vi "Detector Raw Image.vi"(8 "error in (no error)":errorcluster) -> (0 "error out":errorcluster)   [LabVIEW 2018]
uses:
  SesWrapper/SesWrapper.lvlib
panel:
  in  "stop":bool
  out "Camera Image":u8[][](graph)
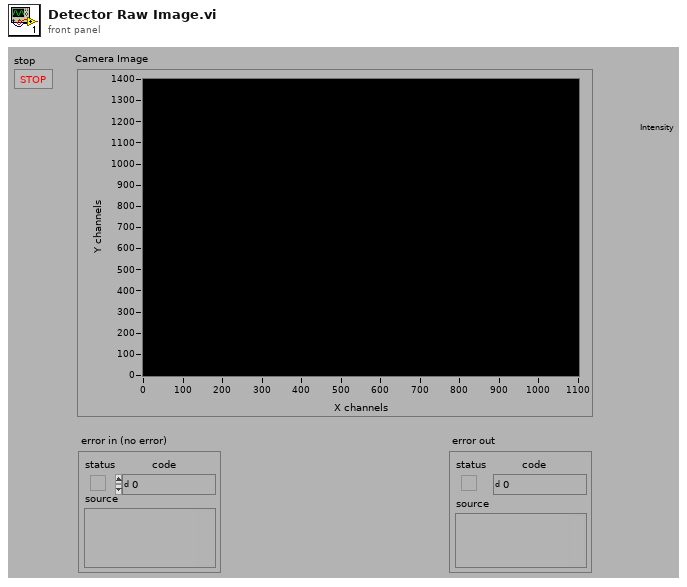
[diagram p1: front panel]
types:
  T1 = cluster{"timerControlled_":u8, "@dummy control@":i8, "@dummy control@":i8, "@dummy control@":i8, "xChannels_":i32, "yChannels_":i32, "maxSlices_":i32, "maxChannels_":i32, "frameRate_":i32, "adcPresent_":u8, "discPresent_":u8}
  T2 = cluster{"timerControlled_":u8, "xChannels_":i32, "yChannels_":i32, "maxSlices_":i32, "maxChannels_":i32, "frameRate_":i32, "adcPresent_":u8, "discPresent_":u8}
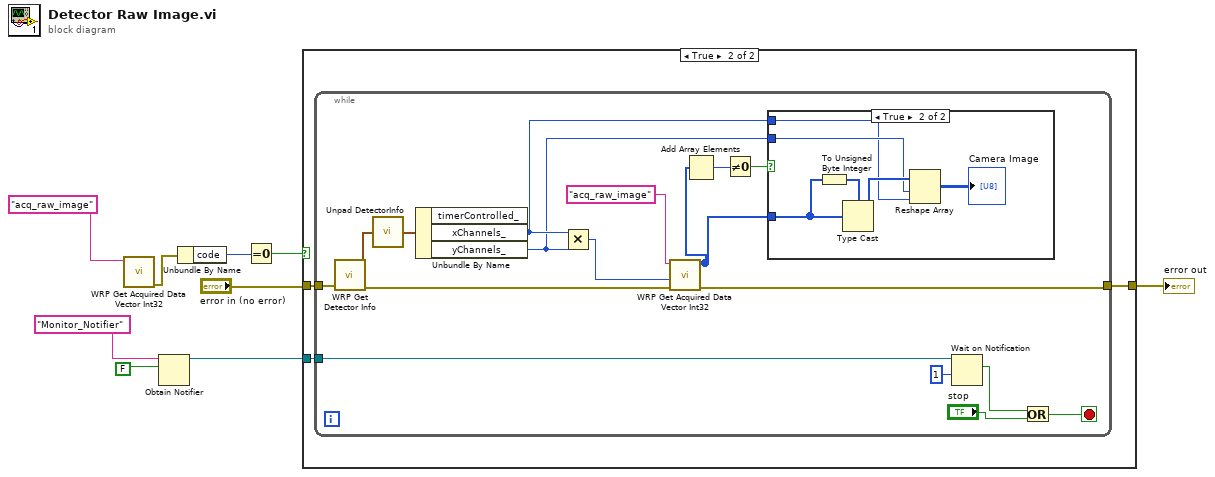
[diagram p0: block diagram]
diagram:
  n1 = call "WRP Get Acquired Data Vector Int32.vi"("parameter"="acq_raw_image") -> ("error out"=w5:errorcluster)  [unwired: 7 in, 3 out]
  n2 = Obtain Notifier(name (unnamed)="Monitor_Notifier", notification data type=FALSE) -> (notifier out=w7:refnum<notifier>)  [unwired: 2 in, 2 out]
  n3 = Unbundle By Name(w5) -> ("code"=w3:i32)
  n4 = Equal To 0?(x=w3) -> (x = 0?=w4:bool)
  n5 = case shown="True" w4 {
    tunnel: [w10 w13] -> w9
    tunnel: w7 -> [_ w12]
    tunnel: "error in (no error)" -> [w10 w11]
    frame False {
    }
    frame True {
      n6 = while {
        tunnel: [w29] -> w13
        tunnel: w11 -> [w20]
        tunnel: w12 -> [w19]
        stop <- w15 stop-if-true
        n7 = call "WRP Get Detector Info.vi"("error in (no error)"=w20) -> ("error out"=w28:errorcluster, "value"=w22:T1)  [unwired: 8 in, 1 out]
        n8 = call "Unpad DetectorInfo.vi"("Detector Info"=w22) -> ("Detector Info out"=w21:T2)
        n9 = Unbundle By Name(w21) -> ("xChannels_"=w27:i32, "yChannels_"=w26:i32)  [unwired: 1 out]
        n10 = Multiply(x=w27, y=w26) -> (x*y=w18:i32)
        n11 = call "WRP Get Acquired Data Vector Int32.vi"("error in (no error)"=w28, "size"=w18, "parameter"="acq_raw_image") -> ("error out"=w29:errorcluster, "data"=w25:i32[])  [unwired: 5 in, 2 out]
        n12 = Add Array Elements(numeric array=w25) -> (sum=w23:i32)
        n13 = Not Equal To 0?(x=w23) -> (x != 0?=w24:bool)
        n14 = case shown="True" w24 {
          tunnel: w25 -> [_ w33]
          tunnel: w27 -> [_ w31]
          tunnel: w26 -> [_ w32]
          frame False {
          }
          frame True {
            n15 = To Unsigned Byte Integer(number=w33) -> (unsigned 8bit integer=w34:u8[])
            n16 = Type Cast(type=w34, x=w33) -> (*(type *) &x=w36:u8[])
            n17 = Reshape Array(w36, w32, w31) -> (→"Camera Image":u8[][])
          }
        }
        n18 = Wait on Notification(notifier=w19, timeout in ms (-1)=1) -> (notification=w17:bool)  [unwired: 2 in, 3 out]
        n19 = Or(x=w17, y="stop") -> (x .or. y?=w15:bool)
      }
    }
  }
  "error out" <- w9
